vi "SaveFrame.vi"(8 "Error In":errorcluster, 9 "With labels?":bool, 10 "Frame":T2, 11 "Hand sign":T1) -> (0 "Error Out":errorcluster, 2 "Frame data":string[](array[string]))   [LabVIEW 2017, in "LeapMotion.lvlib"]
uses:
  LeapMotion.lvlib
  TypeDefs/LEAPframe.ctl
  TypeDefs/LEAPhand.ctl
  TypeDefs/LEAPvector.ctl
  TypeDefs/LEAParm.ctl
  TypeDefs/LEAPfinger.ctl
  TypeDefs/LEAPbone.ctl
  TypeDefs/SelectSign.ctl
panel:
  out "size(s)":i32
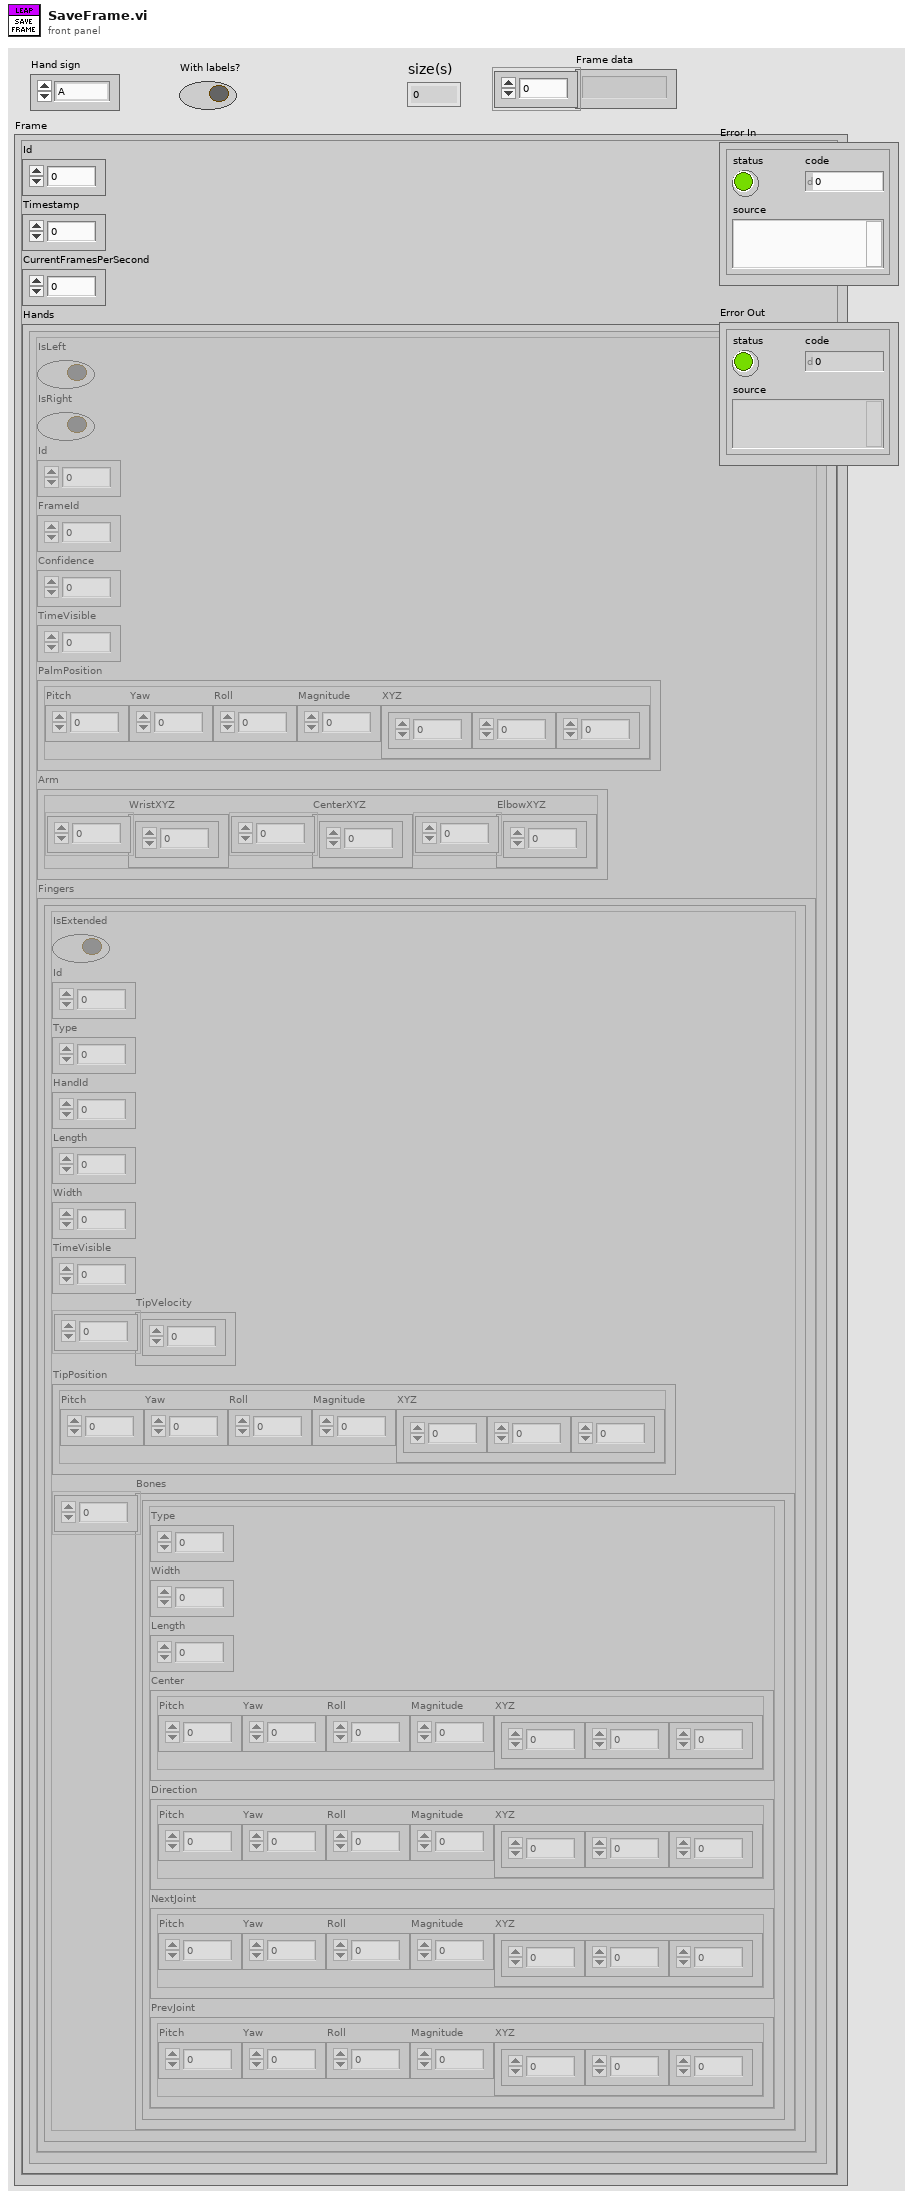
[diagram p1: front panel]
types:
  T1 = typedef "LeapMotion.lvlib/SelectSign.ctl" = enum16{"A", "B", "C", "D", "E", "F", "G", "H", "I", "J", "K", "L", "M", "N", "O", "P", "Q", "R", "S", "T", "U", "V", "W", "X", "Y", "Z"}
  T2 = typedef "LeapMotion.lvlib/LEAPframe.ctl" = cluster{"Id":i64, "Timestamp":i64, "CurrentFramesPerSecond":sgl, "Hands":T3[]}
  T3 = typedef "LeapMotion.lvlib/LEAPhand.ctl" = cluster{"IsLeft":bool, "IsRight":bool, "Id":i32, "FrameId":i64, "Confidence":sgl, "TimeVisible":sgl, "PalmPosition":T4, "Arm":T5, "Fingers":T6[]}
  T4 = typedef "LeapMotion.lvlib/LEAPvector.ctl" = cluster{"Pitch":sgl, "Yaw":sgl, "Roll":sgl, "Magnitude":sgl, "XYZ":sgl[]}
  T5 = typedef "LeapMotion.lvlib/LEAParm.ctl" = cluster{"WristXYZ":sgl[], "CenterXYZ":sgl[], "ElbowXYZ":sgl[]}
  T6 = typedef "LeapMotion.lvlib/LEAPfinger.ctl" = cluster{"IsExtended":bool, "Id":i32, "Type":i32, "HandId":i32, "Length":sgl, "Width":sgl, "TimeVisible":sgl, "TipVelocity":sgl[], "TipPosition":T4, "Bones":T7[]}
  T7 = typedef "LeapMotion.lvlib/LEAPbone.ctl" = cluster{"Type":i32, "Width":sgl, "Length":sgl, "Center":T4, "Direction":T4, "NextJoint":T4, "PrevJoint":T4}
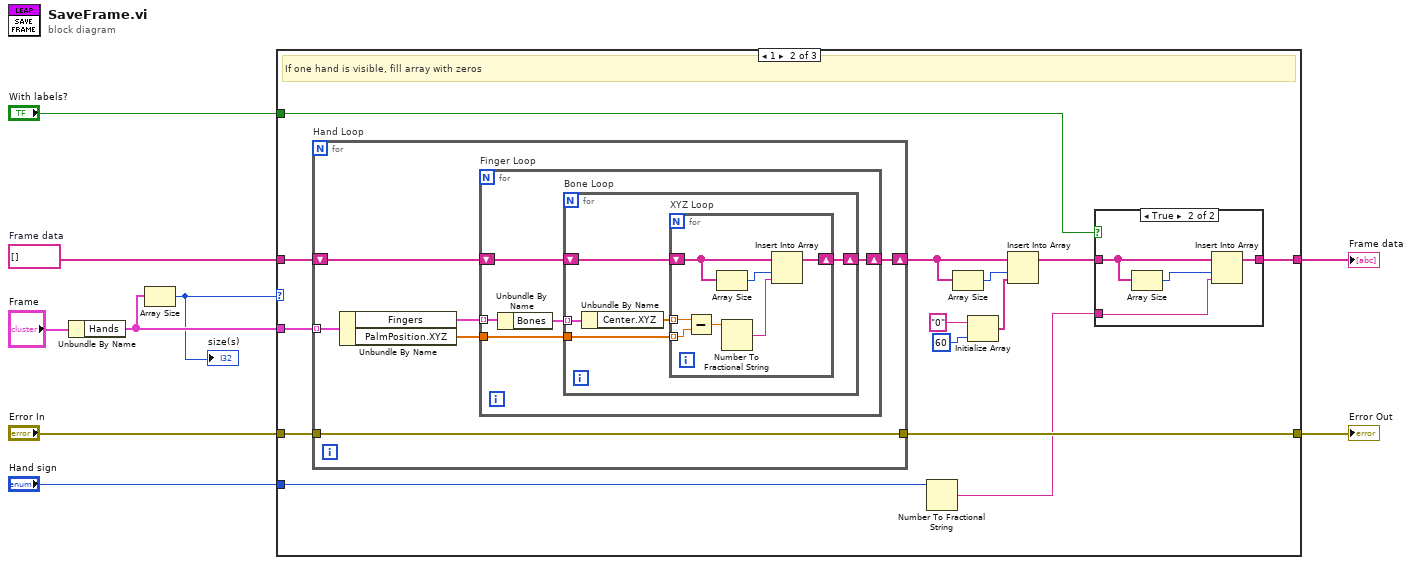
[diagram p0: block diagram]
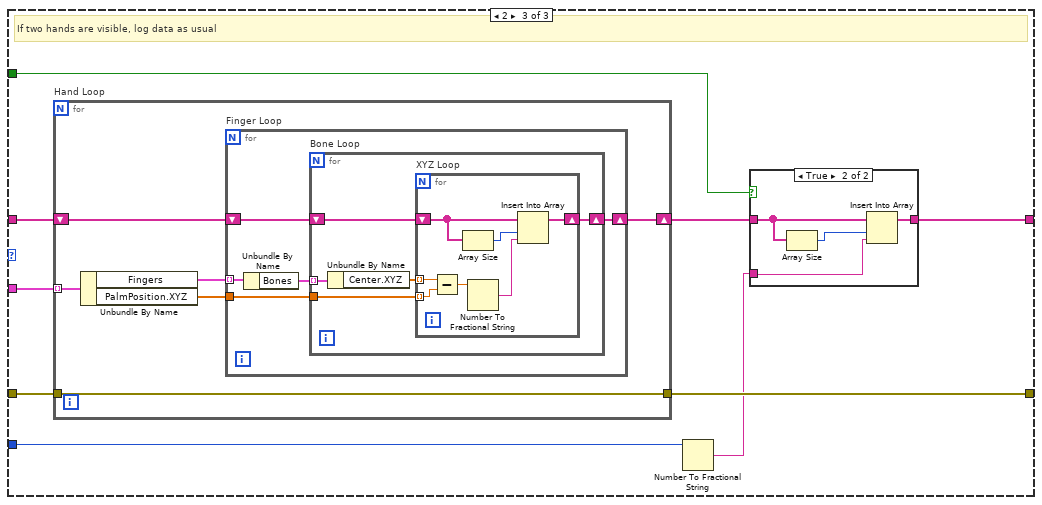
[diagram p4: hidden frame]
diagram:
  w6 = string[] []  # Frame data
  n1 = Unbundle By Name("Frame") -> ("Hands"=w5:T3[])
  n2 = Array Size(array=w5) -> (size(s)=w4:i32)
  "size(s)" <- w4
  n3 = case shown="1" w4 {
    tunnel: "Error In" -> [w11 w25 w62]
    tunnel: [w11 w24 w61] -> w7
    tunnel: w6 -> [w10 w23 w60]
    tunnel: [w10 w21 w57] -> w3
    tunnel: w5 -> [_ w22 w59]
    tunnel: "Hand sign" -> [_ w20 w56]
    tunnel: "With labels?" -> [_ w18 w54]
    frame 0, Default {
      # "If no hands are visible, do not save the frame"
    }
    frame 1 {
      # "If one hand is visible, fill array with zeros"
      n4 = for "Hand Loop" {
        tunnel: w22 -> [w35] mode=indexing
        tunnel: w25 -> [w34]
        tunnel: [w34] -> w24
        shift-right: [w32] -> w14
        shift-left: w23 -> [w33]
        n5 = Unbundle By Name(w35) -> ("Fingers"=w36:T6[], "PalmPosition.XYZ"=w31:sgl[])
        n6 = for "Finger Loop" {
          tunnel: w36 -> [w39] mode=indexing
          shift-right: [w40] -> w32
          shift-left: w33 -> [w41]
          tunnel: w31 -> [w37]
          n7 = Unbundle By Name(w39) -> ("Bones"=w38:T7[])
          n8 = for "Bone Loop" {
            shift-right: [w45] -> w40
            shift-left: w41 -> [w46]
            tunnel: w38 -> [w44] mode=indexing
            tunnel: w37 -> [w42]
            n9 = Unbundle By Name(w44) -> ("Center.XYZ"=w43:sgl[])
            n10 = for "XYZ Loop" {
              shift-right: [w48] -> w45
              shift-left: w46 -> [w49]
              tunnel: w43 -> [w53] mode=indexing
              tunnel: w42 -> [w52] mode=indexing
              n11 = Subtract(x=w53, y=w52) -> (x-y=w51:sgl)
              n12 = Array Size(array=w49) -> (size(s)=w50:i32)
              n13 = Number To Fractional String(number=w51) -> (F-format string=w47:string)  [unwired: 3 in]
              n14 = Insert Into Array(array=w49, index=w50, new element=w47) -> (w48:string[])
            }
          }
        }
      }
      n15 = Number To Fractional String(number=w20) -> (F-format string=w19:string)  [unwired: 3 in]
      n16 = Array Size(array=w14) -> (size(s)=w16:i32)
      n17 = Initialize Array("0" ("element"), 60 ("dimension size")) -> (w15:string[])
      n18 = Insert Into Array(array=w14, index=w16, new element=w15) -> (w13:string[])
      n19 = case shown="True" w18 {
        tunnel: [w26 w29] -> w21
        tunnel: w19 -> [_ w28]
        tunnel: w13 -> [w26 w27]
        frame False {
        }
        frame True {
          n20 = Array Size(array=w27) -> (size(s)=w30:i32)
          n21 = Insert Into Array(array=w27, index=w30, new element=w28) -> (w29:string[])
        }
      }
    }
    frame 2 {
      # "If two hands are visible, log data as usual"
      n22 = for "Hand Loop" {
        tunnel: w59 -> [w72] mode=indexing
        tunnel: w62 -> [w71]
        tunnel: [w71] -> w61
        shift-right: [w69] -> w58
        shift-left: w60 -> [w70]
        n23 = Unbundle By Name(w72) -> ("Fingers"=w73:T6[], "PalmPosition.XYZ"=w68:sgl[])
        n24 = for "Finger Loop" {
          tunnel: w73 -> [w76] mode=indexing
          shift-right: [w77] -> w69
          shift-left: w70 -> [w78]
          tunnel: w68 -> [w74]
          n25 = Unbundle By Name(w76) -> ("Bones"=w75:T7[])
          n26 = for "Bone Loop" {
            shift-right: [w82] -> w77
            shift-left: w78 -> [w83]
            tunnel: w75 -> [w81] mode=indexing
            tunnel: w74 -> [w79]
            n27 = Unbundle By Name(w81) -> ("Center.XYZ"=w80:sgl[])
            n28 = for "XYZ Loop" {
              shift-right: [w85] -> w82
              shift-left: w83 -> [w86]
              tunnel: w80 -> [w90] mode=indexing
              tunnel: w79 -> [w89] mode=indexing
              n29 = Subtract(x=w90, y=w89) -> (x-y=w88:sgl)
              n30 = Array Size(array=w86) -> (size(s)=w87:i32)
              n31 = Number To Fractional String(number=w88) -> (F-format string=w84:string)  [unwired: 3 in]
              n32 = Insert Into Array(array=w86, index=w87, new element=w84) -> (w85:string[])
            }
          }
        }
      }
      n33 = Number To Fractional String(number=w56) -> (F-format string=w55:string)  [unwired: 3 in]
      n34 = case shown="True" w54 {
        tunnel: w58 -> [w63 w67]
        tunnel: [w63 w65] -> w57
        tunnel: w55 -> [_ w64]
        frame False {
        }
        frame True {
          n35 = Array Size(array=w67) -> (size(s)=w66:i32)
          n36 = Insert Into Array(array=w67, index=w66, new element=w64) -> (w65:string[])
        }
      }
    }
  }
  "Error Out" <- w7
  "Frame data" <- w3
